vi "Read Nested Actors.vi"(11 "Template in":refnum<class "Template.lvclass">) -> (3 "Nested Actors":T1(c390))   [LabVIEW 2020, in "Template.lvlib" / "Template.lvclass"]
doc: "Returns the nested actors in the application"
uses:
  Template.lvclass
  <vilib>/ActorFramework/Message Enqueuer/Message Enqueuer.lvclass
  Template.lvclass/Template.ctl
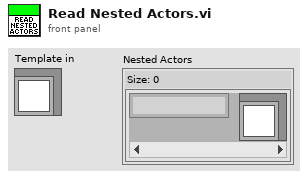
[diagram p1: front panel]
types:
  T1 = map{string, refnum<class "Message Enqueuer.lvclass">}
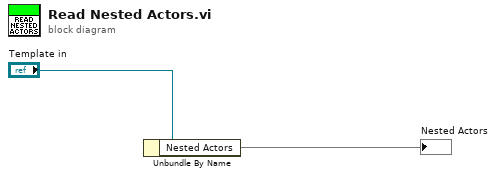
[diagram p0: block diagram]
diagram:
  n1 = Unbundle By Name("Template in") -> ("Nested Actors"=→"Nested Actors":T1)
